vi "MEPmapping.vi"() -> ()   [LabVIEW 2021]
uses:
  <vilib>/numeric/Random Number (Range) I64.vi
  <vilib>/NIOSC/Argument to Float32 Data.vi
  <vilib>/NIOSC/Argument to String Data.vi
  <vilib>/numeric/sub_Random U32.vi
  <vilib>/NIOSC/Generate Error.vi
  <vilib>/NIOSC/Check for Valid String Data.vi
  <vilib>/NIOSC/NI_OSC.lvlib
panel:
  in  "Record":bool
  out "file name (timestamp)":string
  out "XY Graph 2":cluster{"Y":dbl[], "Y":dbl[]}[](graph) caption="XYグラフ"
  out "relative y":dbl
  out "relative x":dbl
  out "all markers info":string
  out "json":string
  out "zdiff":dbl
  out "ydiff":dbl
  out "xdiff":dbl
  in  "stop":bool
  out "XY Graph":cluster{"Y":dbl[], "Y":dbl[]}[](graph) caption="XYグラフ"
  out "波形グラフ":dynamicdata(graph)
  out "数値 2":dbl
  in  "Rep":bool
  out "数値":dbl
  in  "Stop":bool
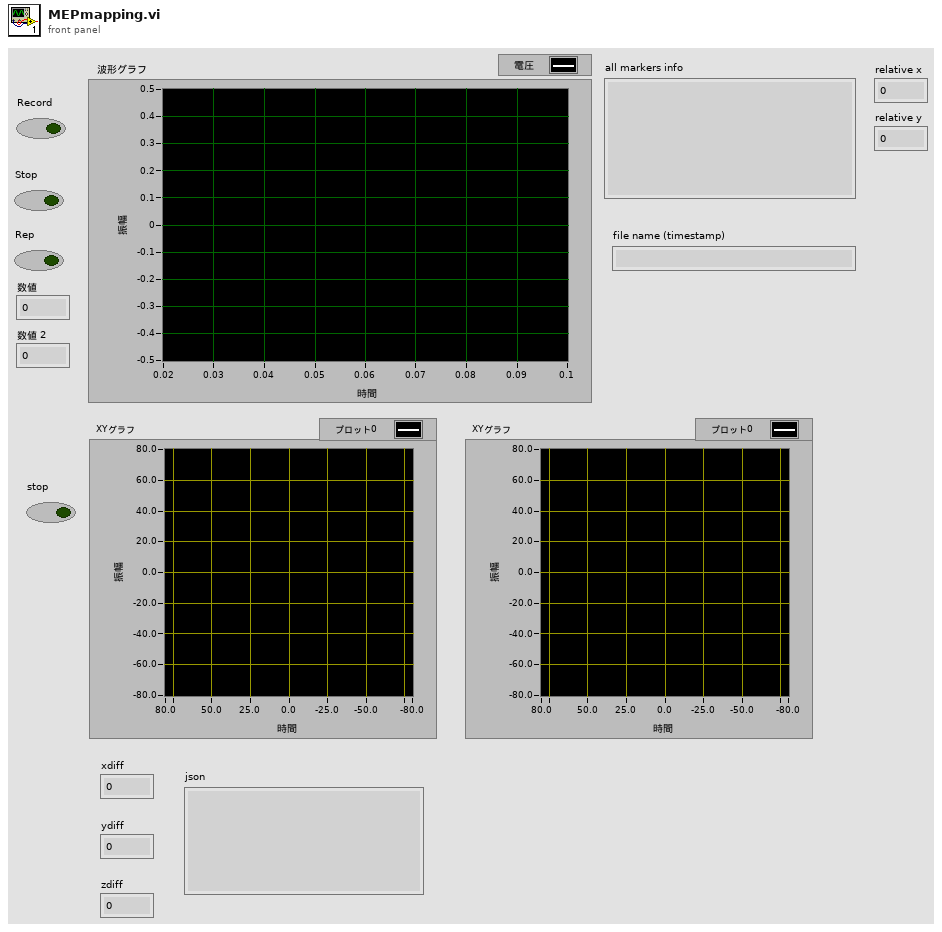
[diagram p1: front panel]
types:
  T1 = typedef "NI_OSC.lvlib/Address Space Node.ctl" = cluster{"parent index":i32, "child indexes":i32[], "address part":string, "method":bool, "data":variant}
  T2 = typedef "NI_OSC.lvlib/Method Dispatching Info.ctl" = cluster{"method address":string, "message":string, "message timetag":u64, "data":variant}
  T3 = typedef "NI_OSC.lvlib/Argument.ctl" = cluster{"argument":string, "type tag":string}
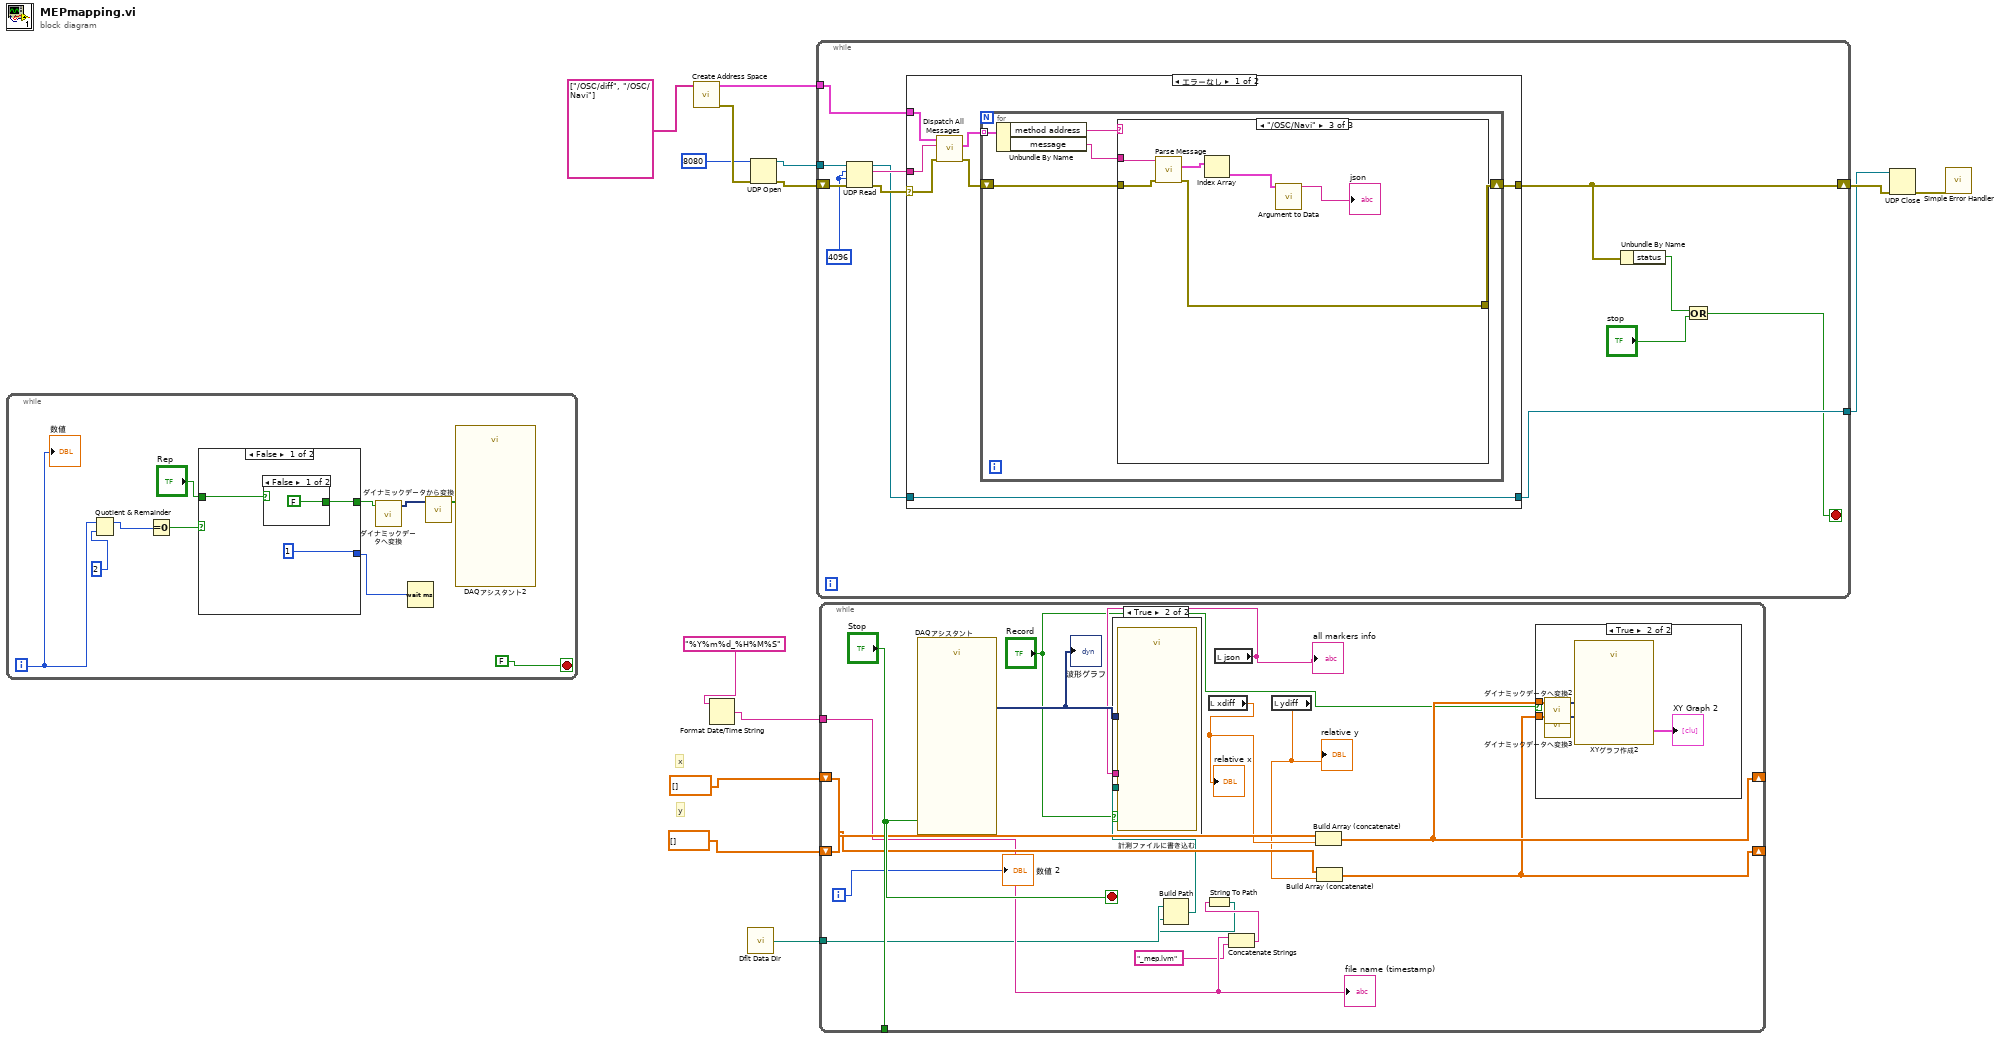
[diagram p0: block diagram]
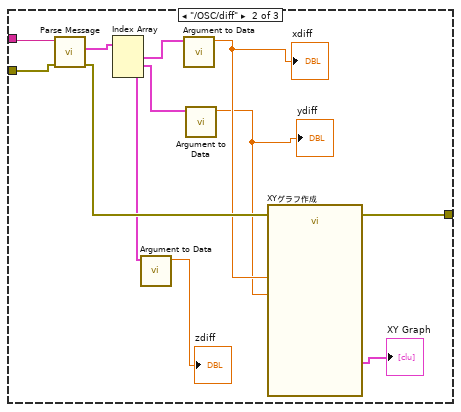
[diagram p3: hidden frame]
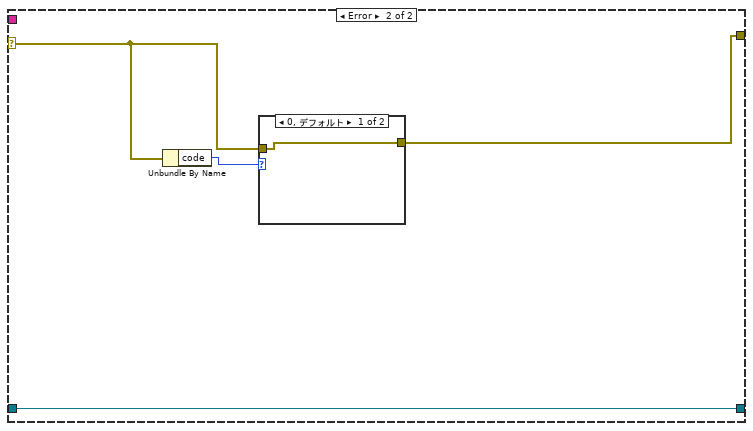
[diagram p4: hidden frame]
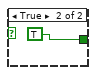
[diagram p6: hidden frame]
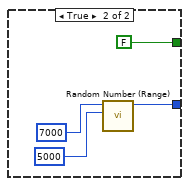
[diagram p7: hidden frame]
diagram:
  # "y"
  # "x"
  n1 = while {
    i -> [w18]
    stop <- FALSE stop-if-true
    n2 = Quotient & Remainder(x=w18, y=2) -> (x-y*floor(x/y)=w24:i32)  [unwired: 1 out]
    n3 = Equal To 0?(x=w24) -> (x = 0?=w16:bool)
    n4 = case shown="FALSE" w16 {
      tunnel: [w27 FALSE] -> w20
      tunnel: [1 w30] -> w19
      tunnel: "Rep" -> [w25 _]
      frame False {
        n5 = case shown="FALSE" w25 {
          tunnel: [FALSE TRUE] -> w27
          frame False {
          }
          frame True {
          }
        }
      }
      frame True {
        n6 = call-poly <vilib>:"Random Number (Range).vi"("lower bound (-100)"=5000, "upper bound (100)"=7000) -> ("number"=w30:i64)  [unwired: 9 in]
      }
    }
    n7 = call "ダイナミックデータへ変換"("Boolean"=w20) -> ("Dynamic Data Type"=w22:dynamicdata)  [unwired: 3 in]
    n8 = Wait (ms)(milliseconds to wait=w19) -> ()  [unwired: 1 out]
    n9 = call "ダイナミックデータから変換"("Dynamic Data Type"=w22) -> ("Array"=w21:bool[])  [unwired: 3 in]
    n10 = call "DAQアシスタント2"("data"=w21) -> ()  [unwired: 17 in, 2 out]
    "数値" <- w18
  }
  n11 = call <vilib>:"Create Address Space.vi"("method addresses"=string[] ["/OSC/diff", "/OSC/Navi"]) -> ("error out"=w13:errorcluster, "address space out"=w9:T1[])  [unwired: 9 in]
  n12 = Format Date/Time String(time format string (%c)="%Y%m%d_%H%M%S") -> (date/time string=w3:string)  [unwired: 2 in]
  n13 = call <vilib>:"Dflt Data Dir.vi"() -> ("App:Default Data Directory"=w1:path)
  n14 = UDP Open(8:w13, 11:8080) -> (port=w11:refnum<k16>, 0:w10:errorcluster)  [unwired: 3 in, 1 out]
  n15 = while {
    tunnel: w11 -> [w45]
    tunnel: w9 -> [w42]
    tunnel: [w39] -> w7
    shift-right: [w38] -> w8
    shift-left: w10 -> [w44]
    stop <- w35 stop-if-true
    w34 = 4096
    n16 = UDP Read(connection ID=w45, max size (548)=w34, timeout ms (25000)=w34, 8:w44) -> (data out=w41:string, error out=w43:errorcluster, 3:w40:refnum<k16>)  [unwired: 2 out]
    n17 = case shown="エラーなし" w43 {
      selector: w43 -> [w49 w77]
      tunnel: w42 -> [w52 _]
      tunnel: w41 -> [w51 _]
      tunnel: w40 -> [w47 w79]
      tunnel: [w47 w79] -> w39
      tunnel: [w46 w76] -> w38
      frame No Error {
        n18 = call <vilib>:"Dispatch All Messages.vi"("error in"=w49, "packet"=w51, "address space in"=w52) -> ("error out"=w48:errorcluster, "method dispatching info"=w50:T2[])  [unwired: 6 in, 1 out]
        n19 = for {
          tunnel: w50 -> [w57] mode=indexing
          shift-right: [w53] -> w46
          shift-left: w48 -> [w54]
          n20 = Unbundle By Name(w57) -> ("method address"=w56:string, "message"=w55:string)
          n21 = case shown="\"/OSC/Navi\"" w56 {
            tunnel: w55 -> [_ w69 w75]
            tunnel: w54 -> [w58 w68 w74]
            tunnel: [w58 w64 w73] -> w53
            frame "FALSE", Default {
            }
            frame "/OSC/diff" {
              n22 = call <vilib>:"Parse Message.vi"("error in"=w68, "message"=w69) -> ("error out"=w64:errorcluster, "arguments"=w62:T3[])  [unwired: 7 in, 1 out]
              n23 = Index Array(array=w62) -> (element #1=w66:T3, element #2=w65:T3, element #3=w63:T3)  [unwired: 3 in]
              n24 = call-poly <vilib>:"Argument to Data.vi"("float32 argument"=w63) -> ("float32 data"=→"zdiff":sgl)  [unwired: 9 in, 1 out]
              n25 = call-poly <vilib>:"Argument to Data.vi"("float32 argument"=w66) -> ("float32 data"=w61:sgl)  [unwired: 9 in, 1 out]
              "xdiff" <- w61
              n26 = call-poly <vilib>:"Argument to Data.vi"("float32 argument"=w65) -> ("float32 data"=w60:sgl)  [unwired: 9 in, 1 out]
              "ydiff" <- w60
              n27 = call "XYグラフ作成"("Y Input"=w60, "X Input"=w61) -> ("XY Graph"=→"XY Graph":cluster{"X":dbl[], "Y":dbl[]}[])  [unwired: 8 in, 1 out]
            }
            frame "/OSC/Navi" {
              n28 = call <vilib>:"Parse Message.vi"("error in"=w74, "message"=w75) -> ("error out"=w73:errorcluster, "arguments"=w72:T3[])  [unwired: 7 in, 1 out]
              n29 = Index Array(array=w72) -> (element=w71:T3)  [unwired: 1 in]
              n30 = call-poly <vilib>:"Argument to Data.vi"("string argument"=w71) -> ("string data"=→"json":string)  [unwired: 9 in, 1 out]
            }
          }
        }
      }
      frame Error {
        n31 = Unbundle By Name(w77) -> ("code"=w78:i32)
        n32 = case shown="0, デフォルト" w78 {
          tunnel: w77 -> [w80 w81]
          tunnel: [w80 w81] -> w76
          frame 0, Default {
          }
          frame 56 {
          }
        }
      }
    }
    n33 = Unbundle By Name(w38) -> ("status"=w37:bool)
    n34 = Or(x=w37, y="stop") -> (x .or. y?=w35:bool)
  }
  n35 = while {
    tunnel: ["Stop"] -> _
    shift-right: [w92] -> _
    shift-left: dbl[] [] -> [w96]
    shift-right: [w91] -> _
    shift-left: dbl[] [] -> [w95]
    tunnel: w3 -> [w89]
    tunnel: w1 -> [w86]
    i -> [w97]
    stop <- "Stop" stop-if-true
    n36 = call "DAQアシスタント"("stop (T)"="Stop") -> ("data"=w90:dynamicdata)  [unwired: 16 in, 2 out]
    "波形グラフ" <- w90
    n37 = local read "xdiff"() -> (w94:dbl)
    "relative x" <- w94
    n38 = local read "json"() -> (w83:string)
    "all markers info" <- w83
    n39 = Concatenate Strings(w89, "_mep.lvm") -> (w87:string)
    n40 = String To Path(string=w87) -> (path=w85:path)
    n41 = Build Path(base path=w86, name or relative path=w85) -> (appended path=w84:path)
    n42 = case shown="TRUE" "Record" {
      tunnel: w90 -> [_ w106]
      tunnel: w84 -> [_ w105]
      tunnel: w83 -> [_ w104]
      frame False {
      }
      frame True {
        n43 = call "計測ファイルに書き込む"("Signals"=w106, "Filename"=w105, "Comment"=w104) -> ()  [unwired: 14 in, 3 out]
      }
    }
    n44 = local read "ydiff"() -> (w93:dbl)
    "relative y" <- w93
    n45 = Build Array (concatenate)(w96, w94) -> (w92:dbl[])
    n46 = Build Array (concatenate)(w95, w93) -> (w91:dbl[])
    n47 = case shown="TRUE" "Record" {
      tunnel: w92 -> [_ w102]
      tunnel: w91 -> [_ w100]
      frame False {
      }
      frame True {
        n48 = call "ダイナミックデータへ変換2"("Array"=w102) -> ("Dynamic Data Type"=w101:dynamicdata)  [unwired: 3 in]
        n49 = call "ダイナミックデータへ変換3"("Array"=w100) -> ("Dynamic Data Type"=w99:dynamicdata)  [unwired: 3 in]
        n50 = call "XYグラフ作成2"("Y Input"=w99, "X Input"=w101) -> ("XY Graph"=→"XY Graph 2":cluster{"X":dbl[], "Y":dbl[]}[])  [unwired: 8 in, 1 out]
      }
    }
    "数値 2" <- w97
    "file name (timestamp)" <- w89
  }
  n51 = UDP Close(connection ID=w7, 8:w8) -> (error out=w6:errorcluster)  [unwired: 1 out]
  n52 = call <vilib>:"Simple Error Handler.vi"("error in (no error)"=w6) -> ()  [unwired: 4 in, 5 out]
